vi "Mass Relink.vi"(8 "error in (no error)":errorcluster, 10 "Mass Relink Directory":path, 11 "Test Executive Builder Model in":refnum<class "Test Executive Builder Model.lvclass">) -> (0 "error out":errorcluster, 3 "Test Executive Builder Model out":refnum<class "Test Executive Builder Model.lvclass">)   [LabVIEW 2017, in "Test Executive Builder Model.lvclass"]
uses:
  <vilib>/gpm_packages/@cs/Test-executive-builder/Source/Test Executive Builder Model/Test Executive Builder Model/Test Executive Builder Model.lvclass
  <vilib>/gpm_packages/@cs/Test-executive-builder/Source/Test Executive Builder Model/Test Executive Builder Model/Test Executive Builder Model.lvclass/Test Executive Builder Model.ctl
  <vilib>/gpm_packages/@cs/test-executive/Source/Test Executive/TestExecutive Ref/TestExecutive Ref.lvclass
panel:
  out "Array":string[](array[string])
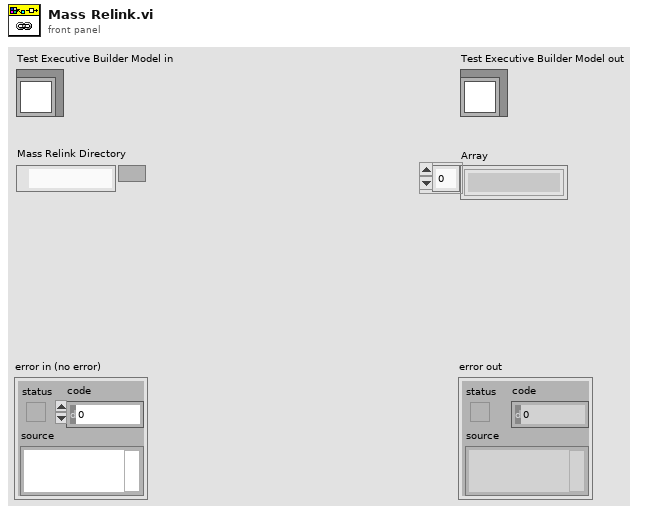
[diagram p1: front panel]
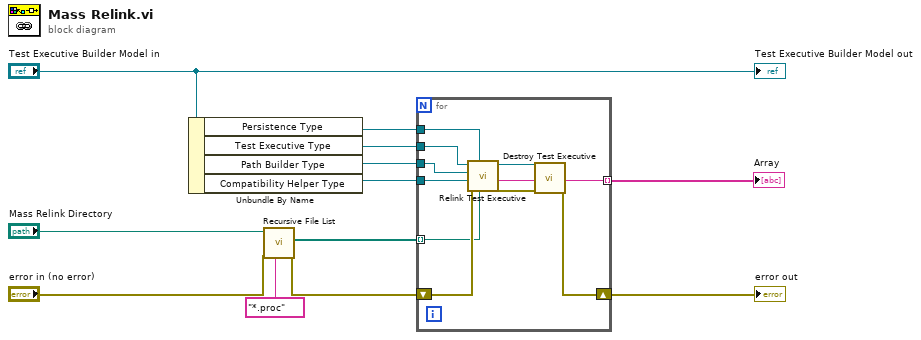
[diagram p0: block diagram]
diagram:
  n1 = Unbundle By Name("Test Executive Builder Model in") -> ("Persistence Type"=w10:refnum<class "IPersist.lvclass">, "Test Executive Type"=w11:refnum<class "ITest Executive.lvclass">, "Path Builder Type"=w9:refnum<class "IPath Builder.lvclass">, "Compatibility Helper Type"=w8:refnum<class "ICompatibility Helper.lvclass">)
  n2 = call <vilib>:"Recursive File List.vi"("pattern"="*.proc", "error in (no error)"="error in (no error)", "Folder Path"="Mass Relink Directory") -> ("error out"=w2:errorcluster, "All Files in Dir"=w4:path[])  [unwired: 4 in, 3 out]
  n3 = for {
    tunnel: w11 -> [w22]
    tunnel: w10 -> [w21]
    tunnel: w9 -> [w20]
    tunnel: w8 -> [w19]
    shift-right: [w15] -> w7
    shift-left: w2 -> [w18]
    tunnel: w4 -> [w14] mode=indexing
    tunnel: [w13] -> w3 mode=indexing
    n4 = call <vilib>:"Relink Test Executive.vi"("File"=w14, "Persistence in"=w21, "error in (no error)"=w18, "Compatibility Helper"=w19, "Path Builder"=w20, "Test Executive"=w22) -> ("error out"=w16:errorcluster, "Return"=w13:string, "Test Executive Ref out"=w17:refnum<data-value>)  [unwired: 2 in, 1 out]
    n5 = call <vilib>:"Destroy Test Executive.vi"("error in (no error)"=w16, "Test Executive Ref"=w17) -> ("error out"=w15:errorcluster)  [unwired: 9 in]
  }
  "error out" <- w7
  "Array" <- w3
  "Test Executive Builder Model out" <- "Test Executive Builder Model in"
